vi "Calculate error and Y0.vi"(6 "ystep":i16, 8 "dx":i16, 9 "dy":i16, 10 "Y0 in":i16, 11 "Error":dbl) -> (2 "Y0 out":i16, 3 "error":dbl)   [LabVIEW 2019]
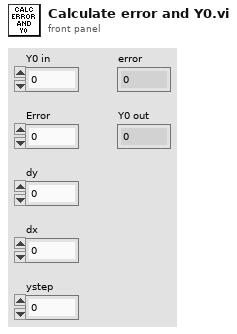
[diagram p1: front panel]
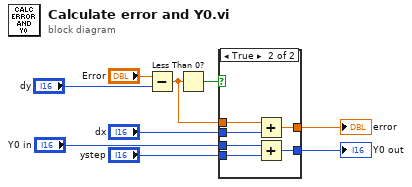
[diagram p0: block diagram]
diagram:
  n1 = Subtract(x="Error", y="dy") -> (x-y=w5:dbl)
  n2 = Less Than 0?(x=w5) -> (x < 0?=w3:bool)
  n3 = case shown="True" w3 {
    tunnel: "Y0 in" -> [w10 w17]
    tunnel: "ystep" -> [_ w16]
    tunnel: [w10 w15] -> w4
    tunnel: w5 -> [w11 w14]
    tunnel: "dx" -> [_ w13]
    tunnel: [w11 w12] -> w7
    frame False {
    }
    frame True {
      n4 = Add(x=w14, y=w13) -> (x+y=w12:dbl)
      n5 = Add(x=w17, y=w16) -> (x+y=w15:i16)
    }
  }
  "error" <- w7
  "Y0 out" <- w4
